vi "niP2P Create Peer to Peer Stream.vi"(0 "writer":refnum<k20>, 5 "reader":refnum<k20>, 7 "enable stream (T)":bool=TRUE, 11 "error in (no error)":errorcluster) -> (4 "stream session":refnum<k20>, 15 "error out":errorcluster)   [LabVIEW 2010]
doc: "Links a writer and reader and creates a stream between them."
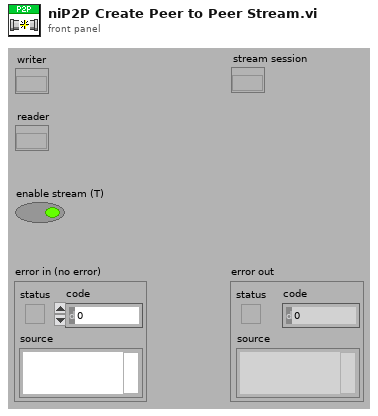
[diagram p1: front panel]
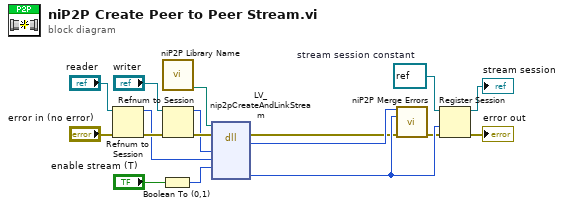
[diagram p0: block diagram]
diagram:
  w4 = refnum<k20> refnum  # stream session constant
  n1 = Refnum to Session(4:"error in (no error)", 7:"reader") -> (0:w16:errorcluster, 3:w10:u64)
  n2 = Boolean To (0,1)(Boolean="enable stream (T)") -> (0, 1=w8:i16)
  n3 = call <vilib>:"niP2P Library Name.vi"() -> ("nip2p libname"=w3:path)  [unwired: 10 in]
  n4 = Refnum to Session(4:w16, 7:"writer") -> (0:w13:errorcluster, 3:w11:u64)
  n5 = dll-call lib="?" fn="LV_nip2pCreateAndLinkStream"(path in=w3, error in=w13, "sourceEndpointHandle"=w11, "sinkEndpointHandle"=w10, "startStream"=w8) -> (error out=w1:errorcluster, "return type"=w6:i32, "streamHandle"=w5:u32)  [unwired: 5 in, 1 out]
  n6 = call <vilib>:"niP2P Merge Errors.vi"("error code"=w6, "stream handle (0)"=w5, "error in"=w1) -> ("error out"=w2:errorcluster)  [unwired: 12 in]
  n7 = Register Session(8:w2, 9:w5, 11:w4) -> (0:→"error out":errorcluster, 3:→"stream session":refnum<k20>)  [unwired: 2 in]
